vi "Configure Current Limit.vi"(7 "Behavior (0: Regulate)":u16(ring) items=["Regulate", "Trip"], 8 "error in (no error)":errorcluster, 9 "Current Limit (0.0 A)":dbl format="%.2g", 10 "Channel (1: Channel 1)":i32(ring)=1 items=["Channel 1"=1, "Channel 2"=2], 11 "VISA resource name":refnum<visa-resource-name>) -> (0 "error out":errorcluster, 3 "VISA resource name out":refnum<visa-resource-name>)   [LabVIEW 2020, in "Template - DC Power.lvlib"]
doc: "Configures over current protection (OCP). Specify the output current limit value and the behavior of the power supply when the output current is greater than or equal to that value."
uses:
  <instrlib>/_Template - DC Power/Template - DC Power.lvlib
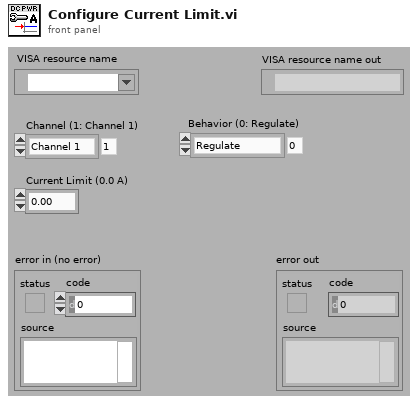
[diagram p1: front panel]
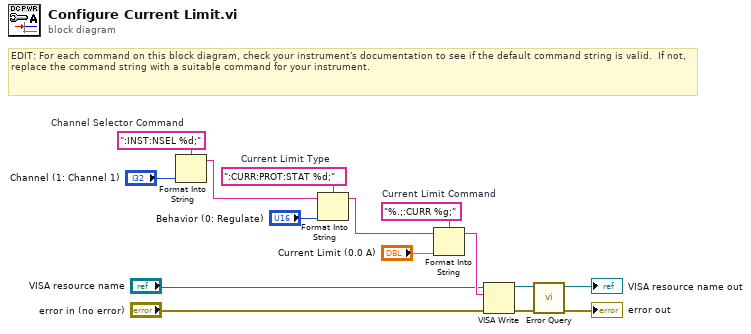
[diagram p0: block diagram]
diagram:
  w4 = ":CURR:PROT:STAT %d;"  # Current Limit Type
  w5 = "%.;:CURR %g;"  # Current Limit Command
  w10 = ":INST:NSEL %d;"  # Channel Selector Command
  # "EDIT: For each command on this block diagram, check your instrument's documentation to see if the default command string is valid.  If not, replace the command string with a suitable command for your instrument."
  n1 = Format Into String(format string=w10, "Channel (1: Channel 1)") -> (resulting string=w3:string)  [unwired: 2 in, 1 out]
  n2 = Format Into String(format string=w4, initial string=w3, "Behavior (0: Regulate)") -> (resulting string=w2:string)  [unwired: 1 in, 1 out]
  n3 = Format Into String(format string=w5, initial string=w2, "Current Limit (0.0 A)") -> (resulting string=w11:string)  [unwired: 1 in, 1 out]
  n4 = VISA Write(VISA resource name="VISA resource name", write buffer=w11, error in (no error)="error in (no error)") -> (VISA resource name out=w13:refnum<visa-resource-name>, error out=w12:errorcluster)  [unwired: 1 out]
  n5 = call <instrlib>:"Error Query.vi"("error in (no error)"=w12, "VISA resource name"=w13) -> ("error out"=→"error out":errorcluster, "VISA resource name out"=→"VISA resource name out":refnum<visa-resource-name>)  [unwired: 6 in, 2 out]
